vi "Scan Engine EtherCAT DS402 Drive Slave.vi"(8 "error in (no error)":errorcluster, 11 "Node Ptr":T1 format="%.0x") -> (0 "error out":errorcluster)   [LabVIEW 2016, in "Scan Engine Custom Device.lvlib"]
uses:
  Scan Engine Custom Device.lvlib
  <vilib>/NI Veristand/Custom Device API/Custom Device Item Ref.ctl
  Globals/Property Strings.vi
  <vilib>/NI Veristand/Custom Device API/Get Item Property (I32).vi
  <vilib>/NI Veristand/Custom Device API/Custom Device API.lvlib
  NationalInstruments.VeriStand.SystemDefinitionAPI
panel:
  out "SW":u16
  out "CW":u16
  out "ToString":string
  in  "Export to XML":bool
  in  "Prepend":bool caption="Prepend slave position to name"
  in  "SHDocVw.IWebBrowser2":refnum<k7>(container)
  in  "Slave Position":u16
  in  "Header":cluster{"Section Name":string}={"Section Name"="EtherCAT Slave"}
  in  "Name":string
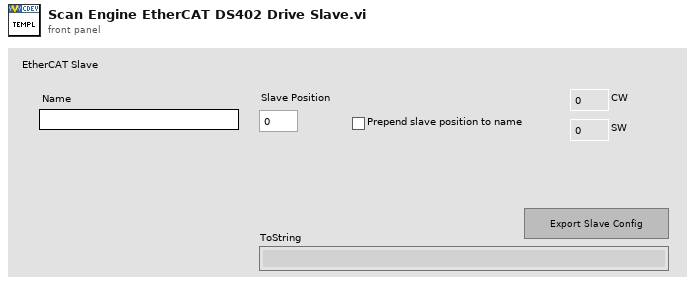
[diagram p1: front panel]
types:
  T1 = typedef "Custom Device API.lvlib/Custom Device Item Ref.ctl" = u64
  T2 = typedef "Custom Device API.lvlib/Custom Device Commands.ctl" = enum16{"Default", "Item renamed", "Shutdown", "Dynamic button pressed"}
  T3 = typedef "Custom Device API.lvlib/Custom Device Pointer.ctl" = refnum<k24>
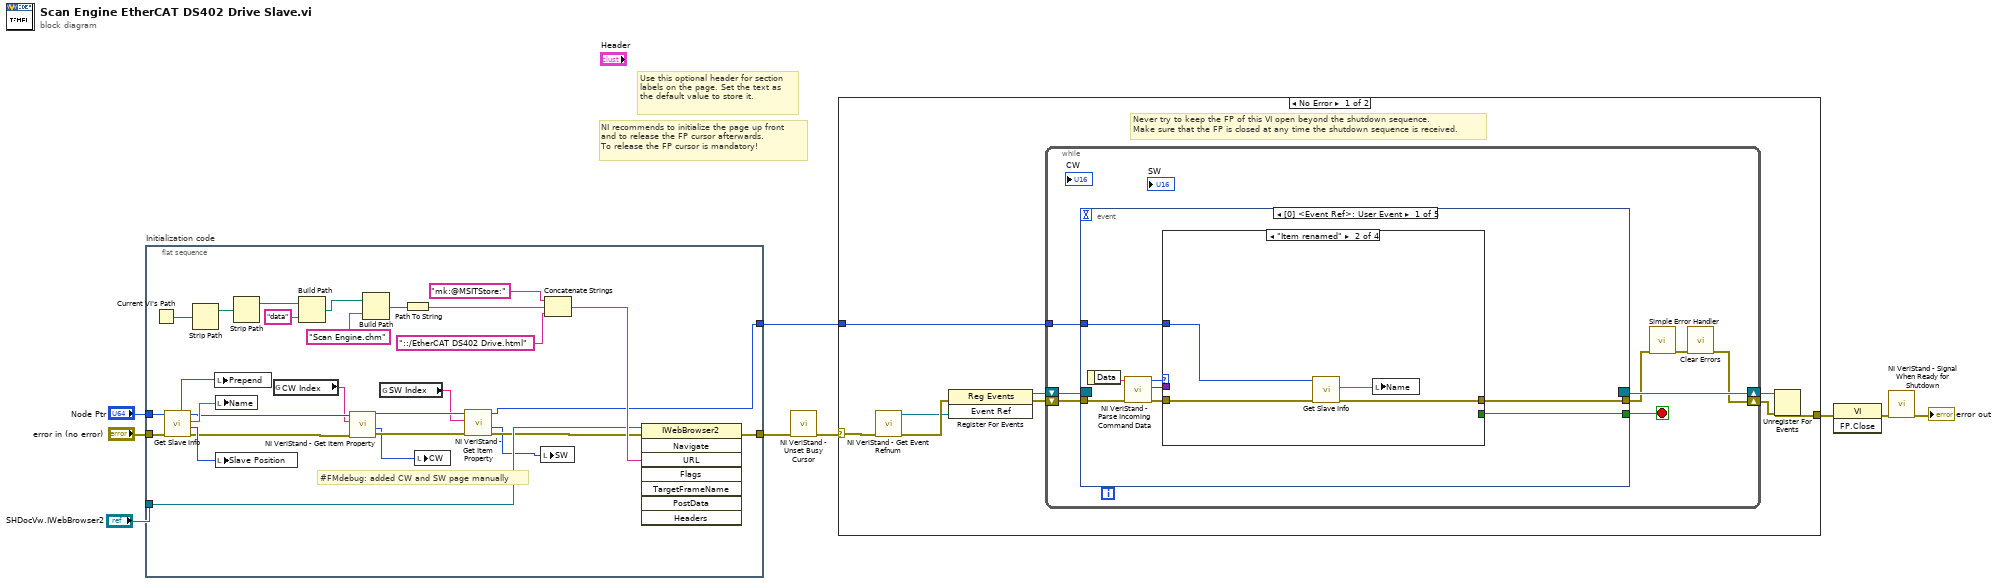
[diagram p0: block diagram]
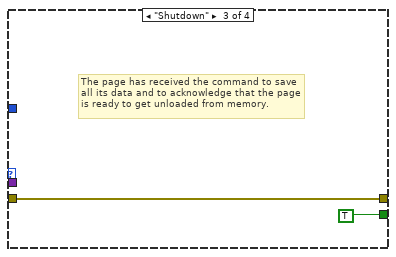
[diagram p3: hidden frame]
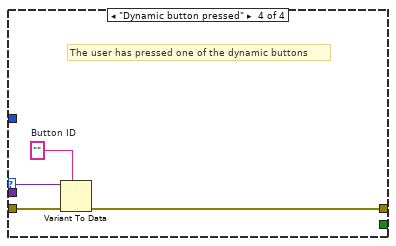
[diagram p4: hidden frame]
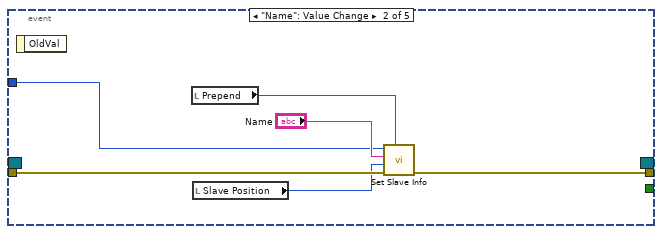
[diagram p5: hidden frame]
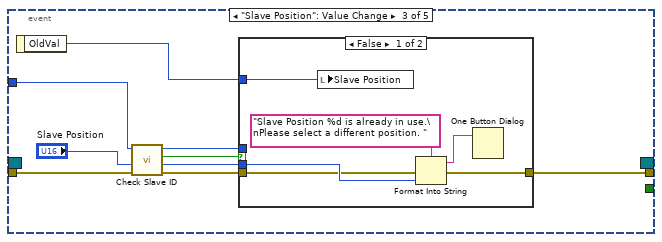
[diagram p6: hidden frame]
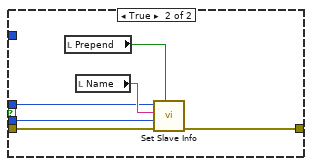
[diagram p7: hidden frame]
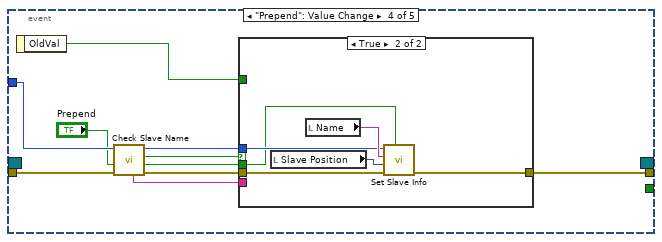
[diagram p8: hidden frame]
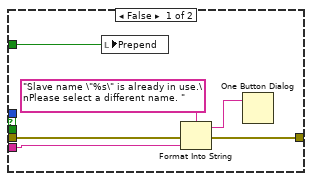
[diagram p9: hidden frame]
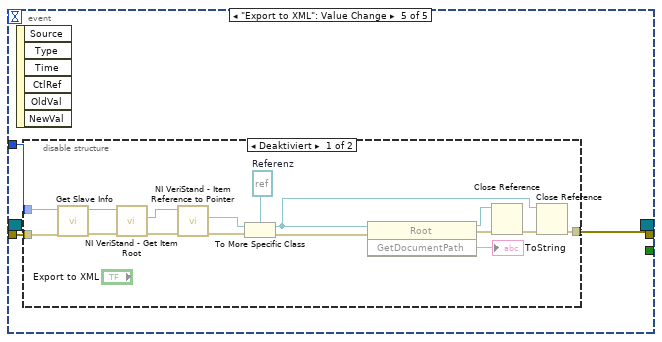
[diagram p10: hidden frame]
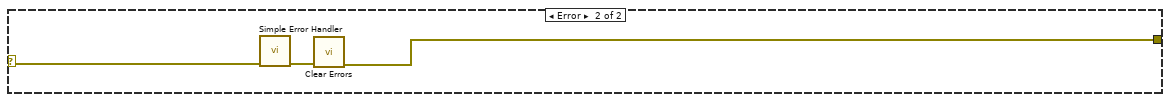
[diagram p12: hidden frame]
diagram:
  # "Use this optional header for section labels on the page. Set the text as the default value to store it."
  # "NI recommends to initialize the page up front\nand to release the FP cursor afterwards.\nTo release the FP cursor is mandatory!"
  n1 = flat-sequence "Initialization code" {
    tunnel: "error in (no error)" -> [w34]
    tunnel: "Node Ptr" -> [w35]
    tunnel: [w24] -> w5
    tunnel: [w13] -> w2
    tunnel: "SHDocVw.IWebBrowser2" -> [w22]
    frame #0 {
      # "#FMdebug: added CW and SW page manually"
      n2 = Current VI's Path() -> (path=w25:path)
      n3 = call "Get Slave Info.vi"("error in (no error)"=w34, "Item Ref in"=w35) -> ("error out"=w19:errorcluster, "Slave #"=w36:u16, "Slave Name"=w37:string, "Item Ref out"=w20:T1, "Prepend"=w21:bool)  [unwired: 5 in]
      n4 = Strip Path(path=w25) -> (stripped path=w26:path)  [unwired: 1 out]
      n5 = local write "Prepend"(w21) -> ()
      n6 = local write "Name"(w37) -> ()
      n7 = local write "Slave Position"(w36) -> ()
      n8 = Strip Path(path=w26) -> (stripped path=w31:path)  [unwired: 1 out]
      n9 = global read "Property Strings.vi" "CW Index"() -> (w15:string)
      n10 = Build Path(base path=w31, name or relative path="data") -> (appended path=w32:path)
      n11 = call-poly <vilib>:"NI VeriStand - Get Item Property.vi"("error in (no error)"=w19, "Property Name"=w15, "Item Ref in"=w20) -> ("error out"=w17:errorcluster, "Value"=w12:i32, "Item Ref out"=w18:T1)  [unwired: 5 in, 1 out]
      n12 = Build Path(base path=w32, name or relative path="Scan Engine.chm") -> (appended path=w29:path)
      n13 = global read "Property Strings.vi" "SW Index"() -> (w14:string)
      n14 = Path To String(path=w29) -> (string=w28:string)
      n15 = local write "CW"(w12) -> ()
      n16 = call-poly <vilib>:"NI VeriStand - Get Item Property.vi"("error in (no error)"=w17, "Property Name"=w14, "Item Ref in"=w18) -> ("error out"=w16:errorcluster, "Value"=w11:i32, "Item Ref out"=w13:T1)  [unwired: 5 in, 1 out]
      n17 = local write "SW"(w11) -> ()
      n18 = Concatenate Strings("mk:@MSITStore:" ("string"), w28, "::/EtherCAT DS402 Drive.html" ("name or relative path")) -> (w23:string)
      n19 = invoke class="IWebBrowser2" method="Navigate"(reference=w22, error in=w16, "URL"=w23) -> (error out=w24:errorcluster)  [unwired: 5 in, 7 out]
    }
  }
  n20 = call <vilib>:"NI VeriStand - Unset Busy Cursor.vi"("error in (no error)"=w5) -> ("error out"=w4:errorcluster)  [unwired: 10 out]
  n21 = case shown="No Error" w4 {
    selector: w4 -> [w38 w144]
    tunnel: [w43 w142] -> w9
    tunnel: w2 -> [w39 _]
    frame No Error {
      # "Never try to keep the FP of this VI open beyond the shutdown sequence.\nMake sure that the FP is closed at any time the shutdown sequence is received."
      n22 = call <vilib>:"NI VeriStand - Get Event Refnum.vi"("error in (no error)"=w38) -> ("error out"=w46:errorcluster, "Event Ref"=w42:refnum<user-event>)  [unwired: 9 out]
      n23 = register-events(error in=w46, w42) -> (reference out=w40:refnum<event-registration>, error out=w41:errorcluster)  [unwired: 1 in]
      n24 = while {
        tunnel: w39 -> [w50]
        shift-right: [w47] -> w44
        shift-left: w41 -> [w53]
        shift-right: [w54] -> w45
        shift-left: w40 -> [w52]
        stop <- w51 stop-if-true
        n25 = event shown="[0] <Event Ref>: User Event" {
          selector: w52 -> [_ _ _ _ _]
          dyn-events: [_ _ _ _ _] -> w54
          timeout: _ -> [_ _ _ _ _]
          tunnel: w53 -> [w62 w77 w82 w108 w125]
          tunnel: [w58 _ _ _ _] -> w51
          tunnel: [w57 w78 w80 w109 w123] -> w49
          tunnel: w50 -> [w56 w76 w84 w107 w124]
          event User Event {
            n26 = event-data() -> ("Data"=w61:string)  [unwired: 1 out]
            n27 = call <vilib>:"NI VeriStand - Parse Incoming Command Data.vi"("error in (no error)"=w62, "Incoming data"=w61) -> ("error out"=w60:errorcluster, "Outgoing data"=w55:variant, "Action"=w59:T2)  [unwired: 7 out]
            n28 = case shown="\"Item renamed\"" w59 {
              tunnel: w60 -> [w63 w67 w68 w73]
              tunnel: [_ _ TRUE _] -> w58
              tunnel: [w63 w66 w68 w70] -> w57
              tunnel: w56 -> [_ w64 _ _]
              tunnel: w55 -> [_ _ _ w72]
              frame "Default", Default {
              }
              frame "Item renamed" {
                n29 = call "Get Slave Info.vi"("error in (no error)"=w67, "Item Ref in"=w64) -> ("error out"=w66:errorcluster, "Slave Name"=w65:string)  [unwired: 5 in, 3 out]
                n30 = local write "Name"(w65) -> ()
              }
              frame "Shutdown" {
                # "The page has received the command to save all its data and to acknowledge that the page is ready to get unloaded from memory."
              }
              frame "Dynamic button pressed" {
                w71 = ""  # Button ID
                # "The user has pressed one of the dynamic buttons"
                n31 = Variant To Data(error in=w73, type=w71, Variant=w72) -> (error out=w70:errorcluster)  [unwired: 1 out]
              }
            }
          }
          event "Name": Value Change {
            n32 = event-data() -> ()  [unwired: 2 out]
            n33 = local read "Prepend"() -> (w74:bool)
            n34 = local read "Slave Position"() -> (w75:u16)
            n35 = call "Set Slave Info.vi"("Prepend"=w74, "error in (no error)"=w77, "Slave #"=w75, "Slave Name"="Name", "Item Ref in"=w76) -> ("error out"=w78:errorcluster)  [unwired: 5 in, 1 out]
          }
          event "Slave Position": Value Change {
            n36 = event-data() -> ("OldVal"=w81:u16)  [unwired: 1 out]
            n37 = call "Check Slave ID.vi"("error in (no error)"=w82, "Slave ID in"="Slave Position", "Item Ref in"=w84) -> ("error out"=w88:errorcluster, "Slave ID out"=w86:u16, "Available?"=w87:bool, "Item Ref out"=w85:T1)  [unwired: 5 in]
            n38 = case shown="False" w87 {
              tunnel: [w90 w100] -> w80
              tunnel: w88 -> [w91 w99]
              tunnel: w85 -> [_ w96]
              tunnel: w86 -> [w93 w98]
              tunnel: w81 -> [w89 _]
              frame False {
                n39 = local write "Slave Position"(w89) -> ()
                n40 = Format Into String(format string="Slave Position %d is already in use.\nPlease select a different position. ", error in=w91, w93) -> (resulting string=w92:string, error out=w90:errorcluster)  [unwired: 1 in]
                n41 = One Button Dialog(message=w92) -> ()  [unwired: 1 in, 1 out]
              }
              frame True {
                n42 = local read "Prepend"() -> (w95:bool)
                n43 = local read "Name"() -> (w97:string)
                n44 = call "Set Slave Info.vi"("Prepend"=w95, "error in (no error)"=w99, "Slave #"=w98, "Slave Name"=w97, "Item Ref in"=w96) -> ("error out"=w100:errorcluster)  [unwired: 5 in, 1 out]
              }
            }
          }
          event "Prepend": Value Change {
            n45 = event-data() -> ("OldVal"=w110:bool)  [unwired: 1 out]
            n46 = call "Check Slave Name.vi"("error in (no error)"=w108, "Prepend in"="Prepend", "Item Ref in"=w107) -> ("error out"=w103:errorcluster, "Prepend out"=w102:bool, "Available?"=w104:bool, "Item Ref out"=w105:T1, "Slave Name"=w101:string)  [unwired: 4 in]
            n47 = case shown="True" w104 {
              tunnel: [w113 w122] -> w109
              tunnel: w103 -> [w114 w121]
              tunnel: w105 -> [_ w119]
              tunnel: w102 -> [_ w118]
              tunnel: w110 -> [w116 _]
              tunnel: w101 -> [w111 _]
              frame False {
                n48 = local write "Prepend"(w116) -> ()
                n49 = Format Into String(format string="Slave name \"%s\" is already in use.\nPlease select a different name. ", error in=w114, w111) -> (resulting string=w112:string, error out=w113:errorcluster)  [unwired: 1 in]
                n50 = One Button Dialog(message=w112) -> ()  [unwired: 1 in, 1 out]
              }
              frame True {
                n51 = local read "Slave Position"() -> (w117:u16)
                n52 = local read "Name"() -> (w120:string)
                n53 = call "Set Slave Info.vi"("Prepend"=w118, "error in (no error)"=w121, "Slave #"=w117, "Slave Name"=w120, "Item Ref in"=w119) -> ("error out"=w122:errorcluster)  [unwired: 5 in, 1 out]
              }
            }
          }
          event "Export to XML": Value Change {
            n54 = event-data() -> ()  [unwired: 7 out]
            n55 = disable-structure shown="Deaktiviert" {
              disable-tunnel: w125 -> [w141 _]
              disable-tunnel: w124 -> [w140 _]
              disable-tunnel: [w135 _] -> w123
              frame Disabled {
                w129 = refnum<k24> refnum  # Referenz
                n56 = call "Get Slave Info.vi"("error in (no error)"=w141, "Item Ref in"=w140) -> ("error out"=w139:errorcluster, "Item Ref out"=w131:T1)  [unwired: 5 in, 3 out]
                n57 = call <vilib>:"NI VeriStand - Get Item Root.vi"("error in (no error)"=w139, "Item Ref in"=w131) -> ("error out"=w132:errorcluster, "Root Ref out"=w128:T1)  [unwired: 6 in, 2 out]
                n58 = call <vilib>:"NI VeriStand - Item Reference to Pointer.vi"("error in (no error)"=w132, "Item Ref in"=w128) -> ("error out"=w134:errorcluster, "Node Pointer"=w127:T3)  [unwired: 6 in, 2 out]
                n59 = To More Specific Class(target class=w129, reference=w127, error in=w134) -> (specific class reference=w130:refnum<k24>, error out=w133:errorcluster)
                n60 = invoke class="Root" method="GetDocumentPath"(reference=w130, error in=w133) -> (reference out=w137:refnum<k24>, error out=w138:errorcluster, "GetDocumentPath"=→"ToString":string)  [unwired: 1 in]
                n61 = Close Reference(reference=w137, error in (no error)=w138) -> (error out=w136:errorcluster)
                n62 = Close Reference(reference=w130, error in (no error)=w136) -> (error out=w135:errorcluster)
              }
              frame Enabled {
              }
            }
          }
        }
        n63 = call <vilib>:"Simple Error Handler.vi"("error in (no error)"=w49) -> ("error out"=w48:errorcluster)  [unwired: 1 in, 7 out]
        n64 = call <vilib>:"Clear Errors.vi"("error in (no error)"=w48) -> ("error out"=w47:errorcluster)  [unwired: 1 in, 5 out]
      }
      n65 = Unregister For Events(event registration refnum=w45, error in=w44) -> (error out=w43:errorcluster)
    }
    frame Error {
      n66 = call <vilib>:"Simple Error Handler.vi"("error in (no error)"=w144) -> ("error out"=w143:errorcluster)  [unwired: 1 in, 7 out]
      n67 = call <vilib>:"Clear Errors.vi"("error in (no error)"=w143) -> ("error out"=w142:errorcluster)  [unwired: 1 in, 5 out]
    }
  }
  n68 = invoke class="VI" method="FP.Close"(error in=w9) -> (error out=w8:errorcluster)  [unwired: 2 in, 2 out]
  n69 = call <vilib>:"NI VeriStand - Signal When Ready for Shutdown.vi"("error in (no error)"=w8) -> ("error out"=→"error out":errorcluster)  [unwired: 10 out]
